vi "RSZVB Set Port Power Generator Offset.vi"(5 "Generator Number (1)":i32=1, 6 "Offset Parameter (1: Add Channel Power)":i32(ring)=1 items=["Only", "Add Channel Power"], 7 "Port Power Offset (0)":dbl format="%^.3e", 8 "error in (no error)":errorcluster {"code" format="%.0x"}, 9 "Port Number (1)":i32=1, 10 "Channel (1)":i32=1, 11 "VISA session":refnum<visa-resource-name>) -> (0 "error out":errorcluster {"code" format="%.0x"}, 3 "dup VISA session":refnum<visa-resource-name>)   [LabVIEW 2011]
doc: "This VI defines the power of an external generator or its power offset relative to the channel power. \n\nNote(s):\n\n(1) This VI is available only on R&S ZVA instrument.\n\nRemote-control command(s):\nSOURce<Ch>:POWer<Pt>:GENerator<Gen>:OFFSet <numeric_value>, ONLY | CPADd"
uses:
  _utility/RSZVB Global Data.vi
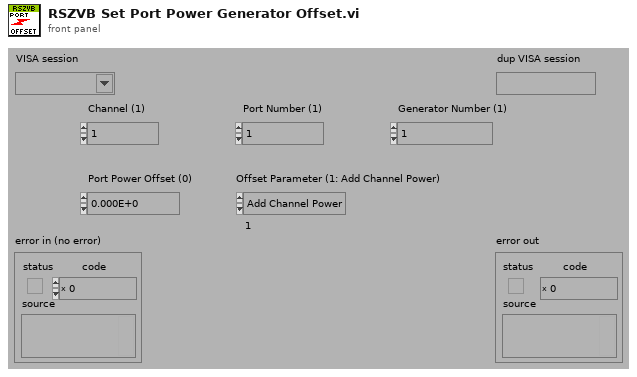
[diagram p1: front panel]
types:
  T1 = cluster{"Error Checking (T: On)":bool, "Installed Options":string[], "Data Valid?":bool, "Ports":i32, "Model":string[], "Option Checking (T: On)":bool}[]
  T2 = cluster{"Error Checking (T: On)":bool, "Installed Options":string[], "Data Valid?":bool, "Ports":i32, "Model":string[], "Option Checking (T: On)":bool}
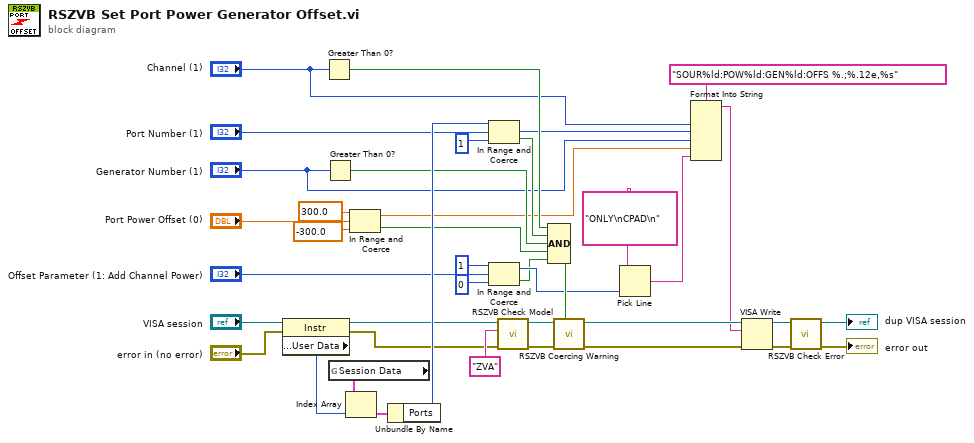
[diagram p0: block diagram]
diagram:
  n1 = property class="Instr"(reference="VISA session", error in="error in (no error)") -> (reference out=w2:refnum<visa-resource-name>, error out=w1:errorcluster, "General Settings:User Data"=w28:u32)
  n2 = Greater Than 0?(x="Channel (1)") -> (x > 0?=w31:bool)
  n3 = Greater Than 0?(x="Generator Number (1)") -> (x > 0?=w9:bool)
  n4 = global read "RSZVB Global Data.vi" "Session Data"() -> (w29:T1)
  n5 = Index Array(array=w29, index=w28) -> (element=w30:T2)
  n6 = In Range and Coerce(upper limit=300.0, x="Port Power Offset (0)", lower limit=-300.0) -> (coerced(x)=w7:dbl, In Range?=w10:bool)
  n7 = Unbundle By Name(w30) -> ("Ports"=w26:i32)
  n8 = In Range and Coerce(upper limit=w26, x="Port Number (1)", lower limit=1) -> (coerced(x)=w24:i32, In Range?=w34:bool)
  n9 = In Range and Coerce(upper limit=1 ("lower limit"), x="Offset Parameter (1: Add Channel Power)", lower limit=0) -> (coerced(x)=w22:i32, In Range?=w11:bool)
  n10 = call "RSZVB Check Model.vi"("error in (no error)"=w1, "Model"="ZVA" ("Options"), "VISA session"=w2) -> ("error out"=w3:errorcluster, "dup VISA session"=w4:refnum<visa-resource-name>)  [unwired: 7 in]
  n11 = Compound Arithmetic op=AND(w31, w34, w9, w10, w11) -> (w33:bool)
  n12 = call "RSZVB Coercing Warning.vi"("In Range?"=w33, "error in (no error)"=w3, "VISA session"=w4) -> ("error out"=w37:errorcluster, "dup VISA session"=w38:refnum<visa-resource-name>)  [unwired: 7 in]
  n13 = Pick Line(multi-line string="ONLY\nCPAD\n", line index=w22) -> (output string=w6:string)  [unwired: 1 in]
  n14 = Format Into String(format string="SOUR%ld:POW%ld:GEN%ld:OFFS %.;%.12e,%s", "Channel (1)", w24, "Generator Number (1)", w7, w6) -> (resulting string=w32:string)  [unwired: 2 in, 1 out]
  n15 = VISA Write(VISA resource name=w38, write buffer=w32, error in (no error)=w37) -> (VISA resource name out=w35:refnum<visa-resource-name>, error out=w36:errorcluster)  [unwired: 1 out]
  n16 = call "RSZVB Check Error.vi"("error in (no error)"=w36, "VISA session"=w35) -> ("error out"=→"error out":errorcluster, "dup VISA session"=→"dup VISA session":refnum<visa-resource-name>)  [unwired: 8 in]
